vi "completeReceiveAllHealthAndStatus.vi"(8 "error in (no error)":errorcluster, 11 "RTHealthAndStatus in":refnum<class "RTHealthAndStatus.lvclass">) -> (0 "error out":errorcluster, 2 "Data":u32[](array[numeric]), 3 "RTHealthAndStatus out":refnum<class "RTHealthAndStatus.lvclass">)   [LabVIEW 2016, in "RTHealthAndStatus.lvlib" / "RTHealthAndStatus.lvclass"]
uses:
  RTHealthAndStatus.lvclass
  RTHealthAndStatus.lvclass/RTHealthAndStatus.ctl
  Common_RT_FPGA/IReadU32FIFO/IReadU32FIFO.lvclass
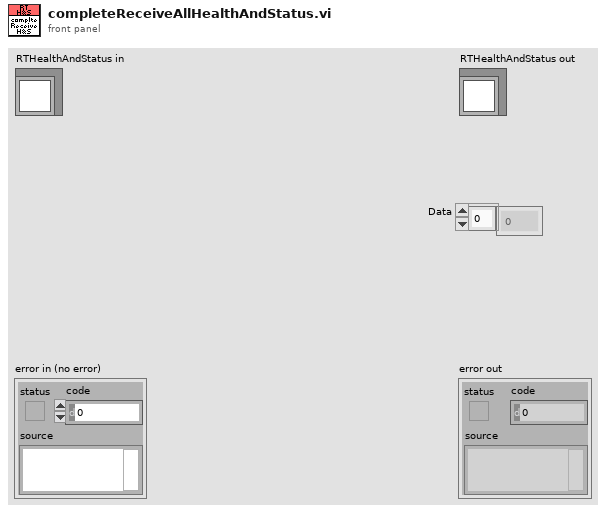
[diagram p1: front panel]
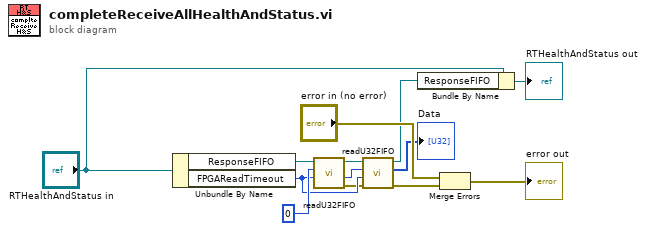
[diagram p0: block diagram]
diagram:
  n1 = Unbundle By Name("RTHealthAndStatus in") -> ("ResponseFIFO"=w8:refnum<class "IReadU32FIFO.lvclass">, "FPGAReadTimeout"=w7:i32)
  n2 = call-dynamic "readU32FIFO.vi"("Timeout"=w7, "NumberOfElements"=u32 0 ("Number of Elements"), "IReadU32FIFO in"=w8) -> ("error out"=w2:errorcluster, "ElementsRemaining"=w6:u32, "IReadU32FIFO out"=w5:refnum<class "IReadU32FIFO.lvclass">)  [unwired: 5 in, 1 out]
  n3 = call-dynamic "readU32FIFO.vi"("error in (no error)"=w2, "Timeout"=w7, "NumberOfElements"=w6, "IReadU32FIFO in"=w5) -> ("error out"=w1:errorcluster, "Data"=→"Data":u32[], "IReadU32FIFO out"=w4:refnum<class "IReadU32FIFO.lvclass">)  [unwired: 4 in, 1 out]
  n4 = Bundle By Name(cluster="RTHealthAndStatus in", "ResponseFIFO"=w4) -> (→"RTHealthAndStatus out":refnum<class "RTHealthAndStatus.lvclass">)
  n5 = Merge Errors("error in (no error)", w1) -> (→"error out":errorcluster)
